vi "Test App Context of Nested App is Set as Direct Parent App.vi"(8 "error in (no error)":errorcluster, 11 "Application Test in":refnum<class "Application Test.lvclass">) -> (0 "error out":errorcluster, 3 "Application Test out":refnum<class "Application Test.lvclass">)   [LabVIEW 2020, in "Application Test.lvclass"]
uses:
  Application Test.lvclass
  C:/Program Files (x86)/National Instruments/LabVIEW 2020/vi.lib/Asteme/LUnit/Test Case.lvclass
  Framework/Application/Application.lvclass
  C:/Users/anton/Documents/GitHub/Triarc-Framework/source/Framework/Process/Process.lvclass
  Framework/Process/Process.lvclass
  Framework/Process/Process.lvclass/Process.ctl
  Framework/Application/Application.lvclass/Application.ctl
  <vilib>/Asteme/LUnit/Test Case.lvclass/Test Case.ctl
  <vilib>/Asteme/LUnit/LUnit Assertion Result.lvclass/LUnit Assertion Result.ctl
  Framework/Process/Protected/SubVIs/Set Context.vi
  Framework/Application/Private/Add Process to Map.vi
  Framework/Process/Protected/Messaging/Enqueue Message.vi
  Framework/Process/Public/Get Lifecycle State.vi
  <vilib>/Asteme/LUnit/Palette/Pass.vi
  <vilib>/Asteme/LUnit/Palette/Fail.vi
  <vilib>/Asteme/LUnit/Variant to string.vi
  <vilib>/Asteme/LUnit/Set Assertion Type.vi
  Framework/Process/Private/SubVIs/Wait for finish.vi
  Framework/Process/Private/SubVIs/Set Lifecycle State.vi
  <vilib>/Utility/error.llb/Clear Errors.vi
  <vilib>/Asteme/LUnit/Add test result.vi
  <vilib>/Asteme/LUnit/LUnit Write Passed.vi
  <vilib>/Asteme/LUnit/LUnit Get Test Case.vi
  <vilib>/Asteme/LUnit/LUnit Write Message.vi
  <vilib>/Asteme/LUnit/LUnit Write Description.vi
  <vilib>/Asteme/LUnit/LUnit Write Assertion Type.vi
  <vilib>/Asteme/LUnit/Read Test Case Name.vi
  <vilib>/Utility/error.llb/Error Cluster From Error Code.vi
  <vilib>/Asteme/LUnit/Assertion Result/LUnit Get Test Name.vi
  <vilib>/Utility/Data Type/Get Type Information.vi
  <vilib>/Utility/LVClass/Get LV Class Name.vi
  <vilib>/Asteme/LUnit/LUnit Assertion Result.lvclass
  <vilib>/Asteme/LUnit/Test Case.lvclass
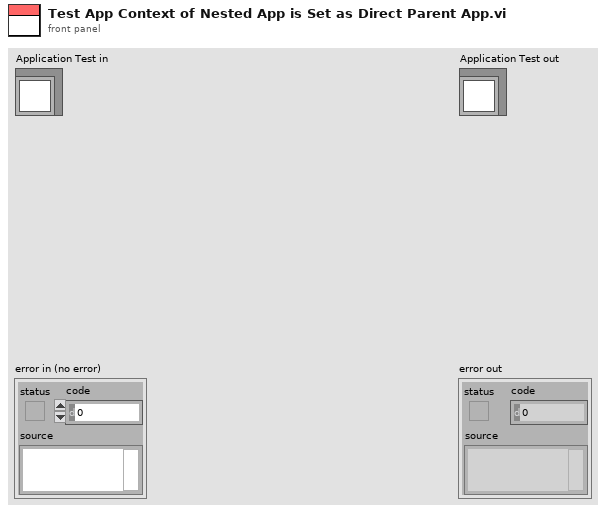
[diagram p1: front panel]
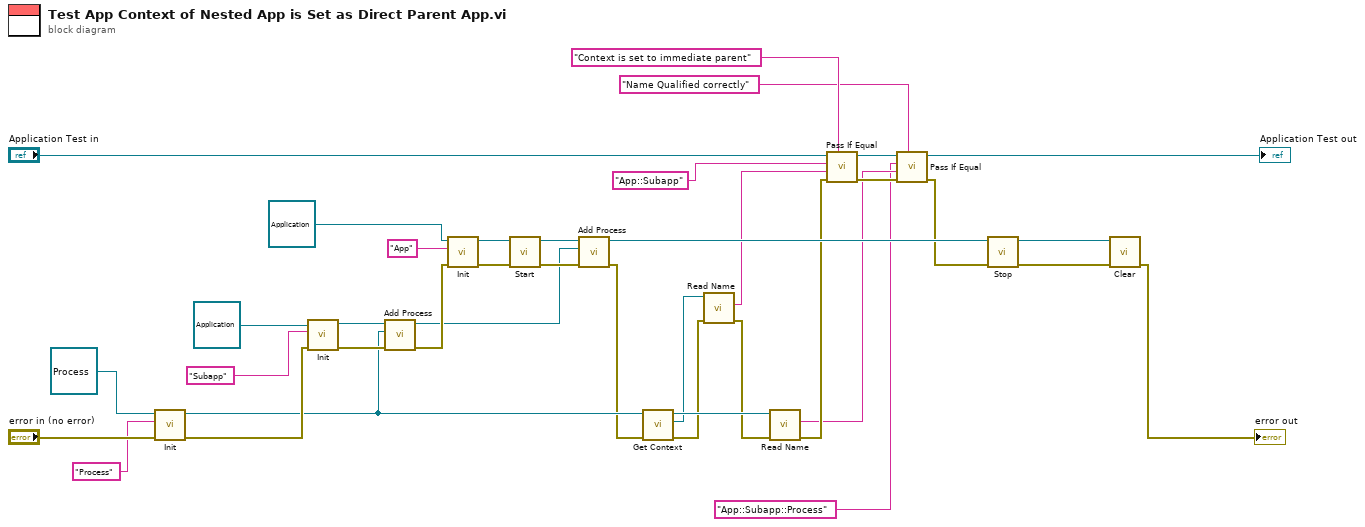
[diagram p0: block diagram]
diagram:
  n1 = call-dynamic "Init.vi"("error in (no error)"="error in (no error)", "Name"="Process", "Process In"=refnum<class "Process.lvclass"> refnum) -> ("error out"=w17:errorcluster, "Process Out"=w16:refnum<class "Process.lvclass">)  [unwired: 7 in]
  n2 = call-dynamic "Init.vi"("error in (no error)"=w17, "Name"="Subapp", "Process In"=refnum<class "Application.lvclass"> refnum ("Application.lvclass")) -> ("error out"=w22:errorcluster, "Process Out"=w23:refnum<class "Application.lvclass">)  [unwired: 7 in]
  n3 = call "Add Process.vi"("error in (no error)"=w22, "Process"=w16, "Rig In"=w23) -> ("error out"=w21:errorcluster, "Rig Out"=w14:refnum<class "Application.lvclass">)  [unwired: 7 in]
  n4 = call-dynamic "Init.vi"("error in (no error)"=w21, "Name"="App", "Process In"=refnum<class "Application.lvclass"> refnum ("Application.lvclass")) -> ("error out"=w37:errorcluster, "Process Out"=w38:refnum<class "Application.lvclass">)  [unwired: 7 in]
  n5 = call "Start.vi"("error in (no error)"=w37, "Process In"=w38) -> ("error out"=w35:errorcluster, "Process Out"=w25:refnum<class "Application.lvclass">)  [unwired: 8 in]
  n6 = call "Add Process.vi"("error in (no error)"=w35, "Process"=w14, "Rig In"=w25) -> ("error out"=w15:errorcluster, "Rig Out"=w28:refnum<class "Application.lvclass">)  [unwired: 7 in]
  n7 = call "Get Context.vi"("error in (no error)"=w15, "Process In"=w16) -> ("error out"=w2:errorcluster, "Context"=w5:refnum<class "Application.lvclass">, "Process Out"=w12:refnum<class "Process.lvclass">)  [unwired: 7 in]
  n8 = call-dynamic "Read Name.vi"("error in (no error)"=w2, "Process In"=w5) -> ("error out"=w1:errorcluster, "Qualified Name"=w4:string)  [unwired: 6 in, 2 out]
  n9 = call-dynamic "Read Name.vi"("error in (no error)"=w1, "Process In"=w12) -> ("error out"=w13:errorcluster, "Qualified Name"=w8:string)  [unwired: 6 in, 2 out]
  n10 = call <vilib>:"Pass If Equal.vi"("Description"="Context is set to immediate parent", "error in (no error)"=w13, "Actual"=w4, "Expected"="App::Subapp" ("Name"), "Test Case In"="Application Test in") -> ("error out"=w10:errorcluster, "Test Case Out"=w34:refnum<class "Application Test.lvclass">)  [unwired: 5 in]
  n11 = call <vilib>:"Pass If Equal.vi"("Description"="Name Qualified correctly", "error in (no error)"=w10, "Actual"=w8, "Expected"="App::Subapp::Process" ("Name"), "Test Case In"=w34) -> ("error out"=w9:errorcluster, "Test Case Out"=→"Application Test out":refnum<class "Application Test.lvclass">)  [unwired: 5 in]
  n12 = call "Stop.vi"("error in (no error)"=w9, "Process In"=w28) -> ("error out"=w31:errorcluster, "Process Out"=w36:refnum<class "Application.lvclass">)  [unwired: 7 in, 1 out]
  n13 = call-dynamic "Clear.vi"("error in (no error)"=w31, "Application In"=w36) -> ("error out"=→"error out":errorcluster)  [unwired: 8 in, 1 out]
